vi "LakeShore336_Controller_v2.vi"() -> ()   [LabVIEW 2020]
uses:
  LabVIEW 2020/instr.lib/Lake Shore 336/Public/Data/Sensor Data (Single Reading).vi
  Users/labpc/Documents/ProbeStation Users Data/Yi Hsun/Yi Hsun LabView Program/SubVIs/Lake Shore 336/Lake Shore 336.lvlib
panel:
  in  "Shield \nRate (D) (%)":dbl format="%.1f"
  in  "Shield \nReset (I)":dbl=20.0 format="%.1f"
  in  "Shield\nGain (P)":dbl=50.0 format="%.1f"
  in  "Stage \nRate (D) (%)":dbl format="%.1f"
  in  "Stage \nReset (I)":dbl=20.0 format="%.1f"
  in  "Stage \nGain (P)":dbl=50.0 format="%.1f"
  out "Shield\nHeater1\nON? (Red)":bool
  out "Stage \nHeater2 \nON? (Red)":bool
  out "Out1 Range":u16(ring) items=["Off", "Low (On)", "Medium", "High"]
  out "Out2 Range":u16(ring) items=["Off", "Low (On)", "Medium", "High"]
  out "Output Sel":u16(ring)=2 items=["1"=1, "2"=2]
  out "Input Sel":u16(ring) items=["A", "B", "C", "D"]
  in  "Run Setup?\nStage Heater":bool
  in  "Stage Setpoint \nRamping Enable":bool=TRUE
  out "Out1 Heater %":dbl format="%.1f"
  out "InB Temp":dbl format="%.4f"
  out "Out1 Setpoint":dbl format="%.5f"
  out "Out2 Heater %":dbl format="%.1f"
  out "InA Temp":dbl format="%.4f"
  out "Out2 Setpoint":dbl format="%.5f"
  out "Out2 Diff. (D)":dbl format="%.1f"
  out "Out2 Int. (I)":dbl=20.0 format="%.1f"
  out "Out2 Prop. (P)":dbl=50.0 format="%.1f"
  out "Out1 Diff. (D)":dbl format="%.1f"
  out "Out1 Int. (I)":dbl=20.0 format="%.1f"
  out "Out1 Prop. (P)":dbl=50.0 format="%.1f"
  out "Probe Arm Temperature":dbl format="%.4f"
  out "Temp vs Time 3":cluster{"Y":dbl[], "Y":dbl[]}[](graph)
  out "Stage Setpoint vs Input X Temp 3":cluster{"Sensor Data":dbl}[](graph)
  out "Shield  vs Time 2":cluster{"Y":dbl[], "Y":dbl[]}[](graph)
  out "Shield Setpoint vs Input X Temp 2":cluster{"Setpoint":dbl, "Sensor Data":dbl}[](graph)
  out "Input Sel 2":u16(ring) items=["A", "B", "C", "D"]
  out "Output Sel2":u16(ring)=2 items=["1"=1, "2"=2]
  in  "Run Setup?\nRadiation Heater":bool
  in  "Shield Heater\nRange":u16(ring) items=["Off", "Low (On)", "Medium", "High"]
  in  "Shield Ramp\nRate (K/min)":dbl=5.0 format="%.1f"
  in  "Shield Setpoint (K)":dbl=290.0 format="%.5f"
  in  "Shield Setpoint \nRamping Enable":bool=TRUE
  out "Stage Temp vs Time":cluster{"Y":dbl[], "Y":dbl[]}[](graph)
  out "Stage Setpoint vs Input X Temp":cluster{"Setpoint":dbl, "Sensor Data":dbl}[](graph)
  in  "Stage Heater\nRange":u16(ring) items=["Off", "Low (On)", "Medium", "High"]
  in  "Stage Ramp\nRate (K/min)":dbl=5.0 format="%.1f"
  in  "Stage Setpoint (K)":dbl=290.0 format="%.5f"
  out "Out4 Setpoint":dbl format="%.5f"
  out "Out3 Setpoint":dbl format="%.5f"
  in  "Sampling (ms) [Min 300ms]":u32=300
  in  "stop":bool
  in  "Serial Configuration 2":T1={"Baud Rate"=57600, "Parity"=1, "Data Bits"=7, "Stop Bits"=10, "Flow Control"=0} {"Flow Control" items=["None", "XON/XOFF", "RTS/CTS", "XON/XOFF & RTS/CTS", "DTR/DSR", "XON/XOFF & DTR/DSR"]; "Stop Bits" items=["1.0"=10, "1.5"=15, "2.0"=20]; "Data Bits" items=["7"=7, "8"=8]; "Parity" items=["None", "Odd", "Even", "Mark", "Space"]; "Baud Rate" items=["300"=300, "600"=600, "1200"=1200, "2400"=2400, "4800"=4800, "9600"=9600, "19200"=19200, "38400"=38400, "57600"=57600]}
  in  "LakeShore 336 esource name":refnum<visa-resource-name>="GPIB0::12::INSTR"
  # "Radiation Shield Controller"
  # "Stage Controller"
  # "Click to run sheild parameter setup -->"
  # "Stage Heater Parameters"
  # "Stage PID Parameters"
  # "Shield Heater Parameters"
  # "Shield PID Parameters"
  # "Stage Heater\nStatus"
  # "Shield Heater\nStatus"
  # "Click to run stage parameter setup -->"
  # "PID\nReadout"
  # "PID\nReadout"
  # "Input & Output\nInformation"
  # "Input Selections\nA - Sample stage,     B - Rad Shield,    \nC - Arm,    D - Disabled"
  # "Output Selections\n1 - Rad Shield,     2 - Sample Stage"
  # "Probe\nArm\nMonitor"
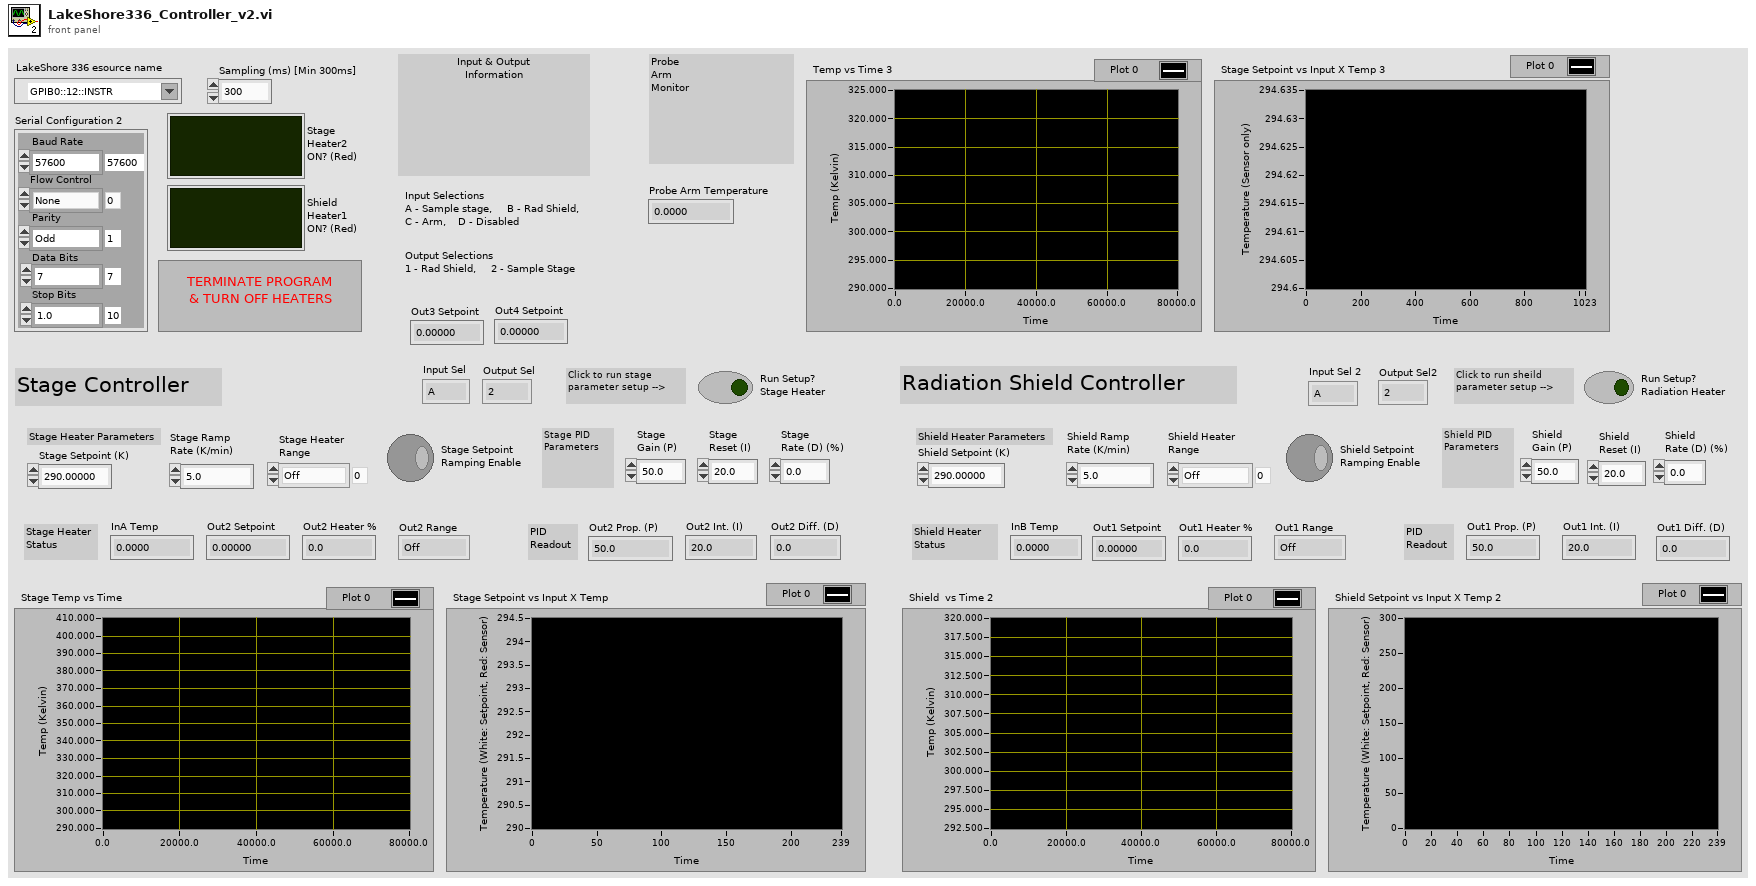
[diagram p1: front panel]
types:
  T1 = cluster{"Baud Rate":u32, "Parity":u16, "Data Bits":u16, "Stop Bits":u16, "Flow Control":u16}
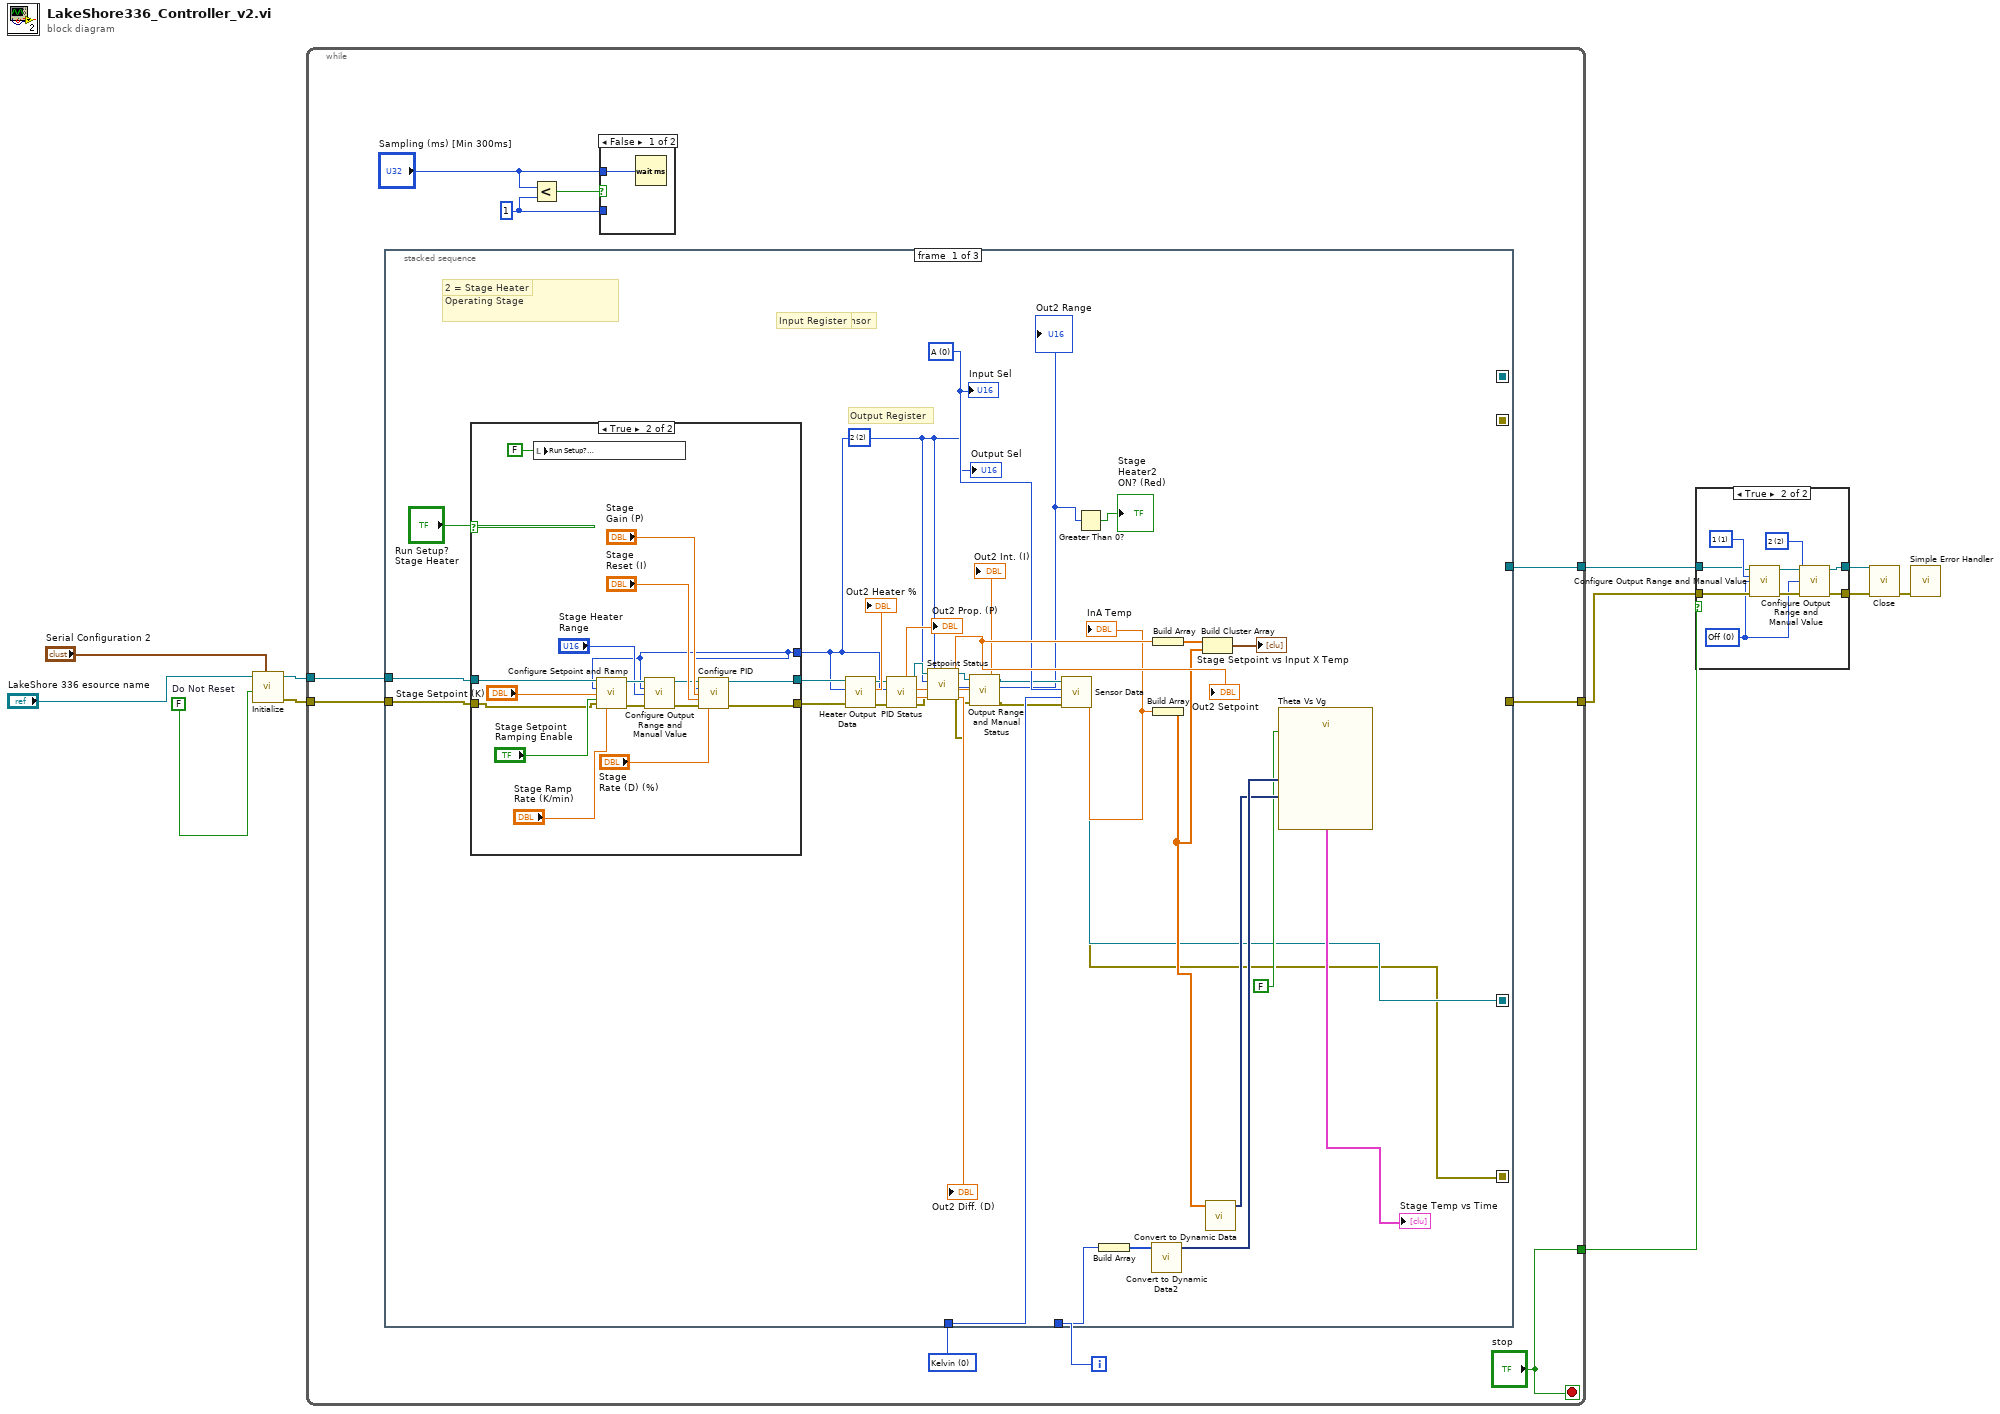
[diagram p0: block diagram]
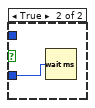
[diagram p3: hidden frame]
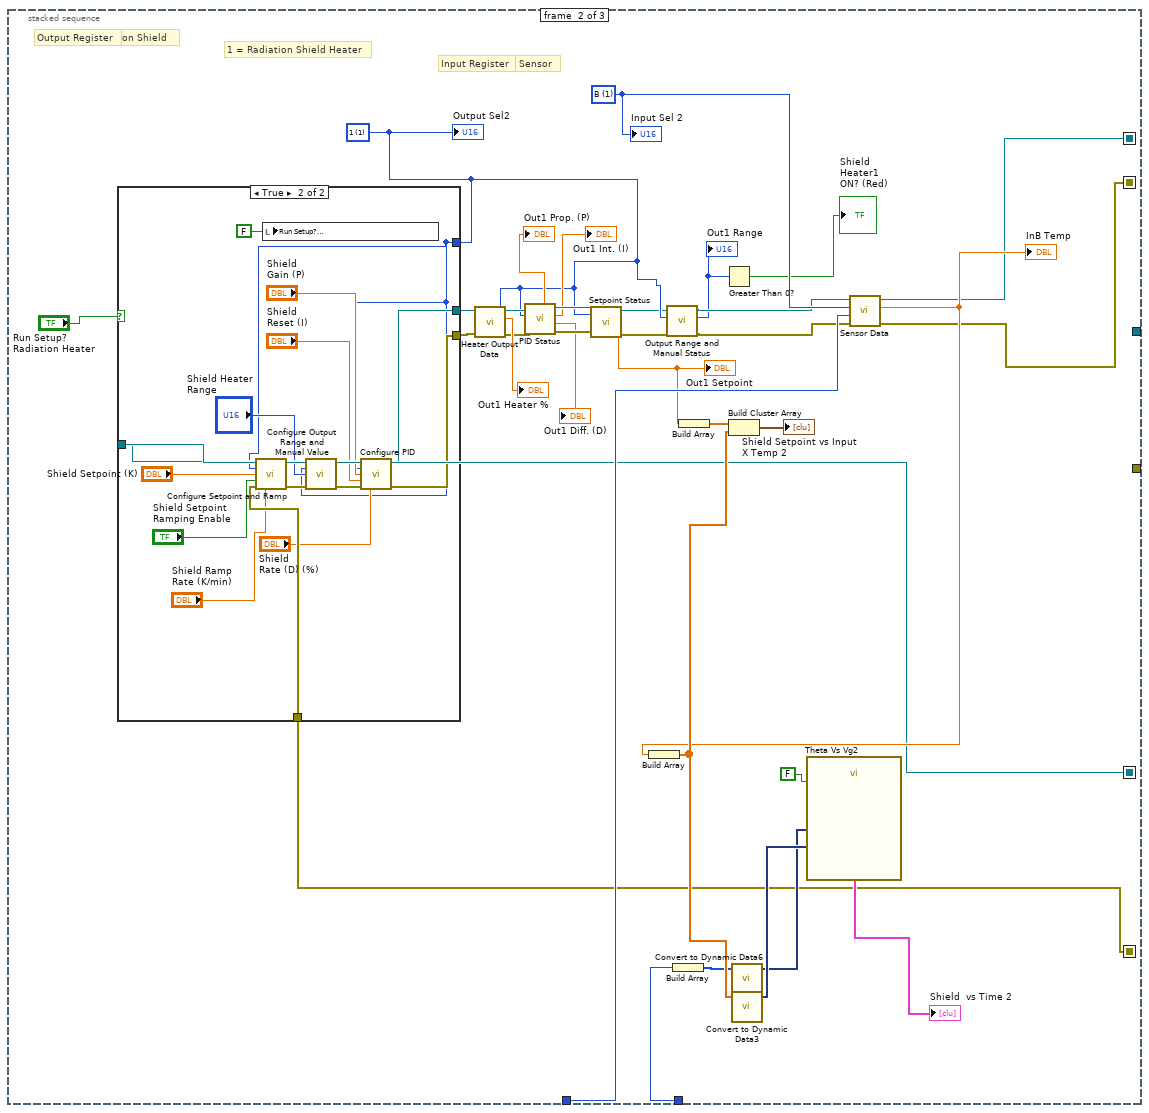
[diagram p5: hidden frame]
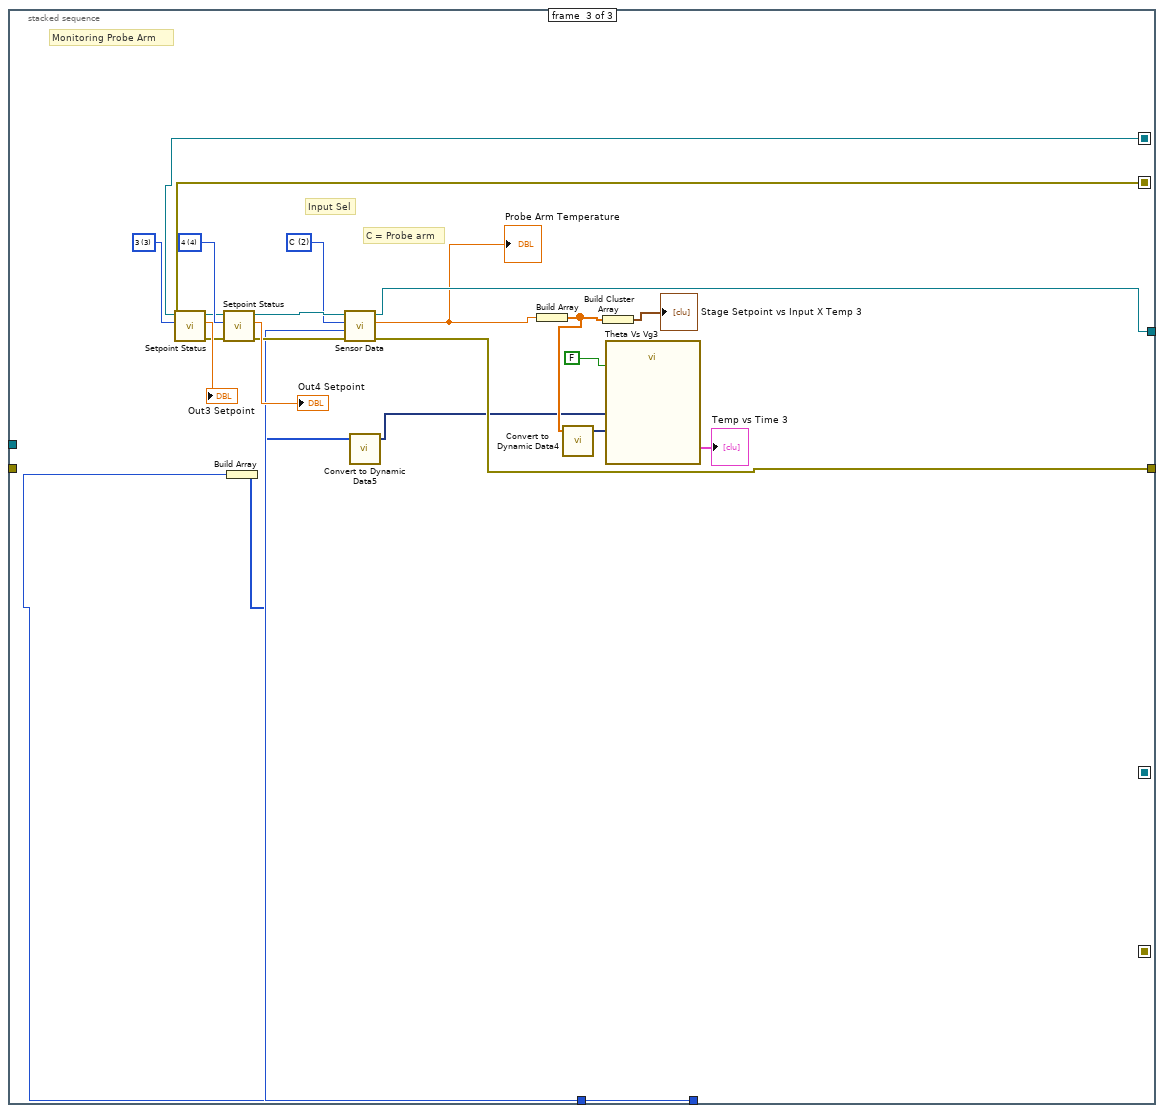
[diagram p7: hidden frame]
diagram:
  w9 = FALSE  # Do Not Reset
  n1 = call "Initialize.vi"("Serial Configuration"="Serial Configuration 2", "Reset (True)"=w9, "VISA resource name"="LakeShore 336 esource name") -> ("error out"=w6:errorcluster, "VISA resource name out"=w7:refnum<visa-resource-name>)  [unwired: 7 in]
  n2 = while {
    tunnel: w7 -> [w21]
    tunnel: w6 -> [w20]
    tunnel: [w19] -> w4
    tunnel: [w18] -> w2
    tunnel: ["stop"] -> w5
    i -> [w14]
    stop <- "stop" stop-if-true
    w13 = u16 0 items=["Kelvin", "Celsius", "Sensor Units"] ("Data Source (0:Kelvin)")
    w16 = u32 1 ("y")
    n3 = stacked-sequence {
      seq-local: [w42 _ _] -> [_ w98 _]
      seq-local: [w41 _ _] -> [_ w97 _]
      seq-local: [_ w96 _] -> [_ _ w147]
      seq-local: [_ w95 _] -> [_ _ w146]
      tunnel: w21 -> [w57 _ _]
      tunnel: w20 -> [w56 _ _]
      tunnel: [_ _ w143] -> w19
      tunnel: [_ _ w142] -> w18
      tunnel: w14 -> [w45 w102 w134]
      tunnel: w13 -> [w43 w104 w138]
      frame #0 {
        w47 = u16 0 items=["A", "B", "C", "D"] ("Input (0:A)\nA - Sample\nB - Rad Shield\nC - Arm\nD - Disabled")
        w26 = u16 2 items=["1"=1, "2"=2] ("Heater Output (1:1)")
        # "A = Stage Sensor"
        # "2 = Stage Heater"
        # "Input Register"
        # "Output Register"
        # "Operating Stage"
        n4 = case shown="True" "Run Setup?\nStage Heater" {
          tunnel: w57 -> [w60 w71]
          tunnel: w56 -> [w59 w70]
          tunnel: [w60 w61] -> w40
          tunnel: [w59 w62] -> w39
          tunnel: w26 -> [_ w65]
          frame False {
          }
          frame True {
            n5 = local write "Run Setup?\nStage Heater"(FALSE ("Run Stage Heater Setup?\nOff / On")) -> ()
            n6 = call "Configure Setpoint and Ramp.vi"("VISA resource name"=w71, "Output's Control Loop (1:1)"=w65, "Setpoint (0.00000)"="Stage Setpoint (K)", "Setpoint Ramping \nEnable (F: Off)"="Stage Setpoint \nRamping Enable", "error in (no error)"=w70, "Ramp Rate (0.0)"="Stage Ramp\nRate (K/min)") -> ("VISA resource name out"=w74:refnum<visa-resource-name>, "error out"=w73:errorcluster)  [unwired: 8 in]
            n7 = call "Configure Output Range and Manual Value.vi"("VISA resource name"=w74, "Output (1:1)"=w65, "Range (0:Off)"="Stage Heater\nRange", "error in (no error)"=w73) -> ("VISA resource name out"=w64:refnum<visa-resource-name>, "error out"=w63:errorcluster)  [unwired: 10 in]
            n8 = call "Configure PID.vi"("VISA resource name"=w64, "Output's Control Loop (1:1)"=w65, "Gain (P) (50.0)"="Stage \nGain (P)", "Reset (I) (20.0)"="Stage \nReset (I)", "error in (no error)"=w63, "Rate (D) (0.0 %)"="Stage \nRate (D) (%)") -> ("VISA resource name out"=w61:refnum<visa-resource-name>, "error out"=w62:errorcluster)  [unwired: 8 in]
          }
        }
        n9 = call "Heater Output Data.vi"("error in (no error)"=w39, "Heater Output (1:1)"=w26, "VISA resource name"=w40) -> ("error out"=w36:errorcluster, "Output Value"=→"Out2 Heater %":dbl, "VISA resource name out"=w37:refnum<visa-resource-name>)  [unwired: 6 in]
        n10 = call "PID Status.vi"("error in (no error)"=w36, "Output's Control Loop (1:1)"=w26, "VISA resource name"=w37) -> ("error out"=w32:errorcluster, "Rate (D)"=→"Out2 Diff. (D)":dbl, "Reset (I)"=→"Out2 Int. (I)":dbl, "VISA resource name out"=w31:refnum<visa-resource-name>, "Gain (P)"=→"Out2 Prop. (P)":dbl)  [unwired: 4 in]
        n11 = call "Setpoint Status.vi"("error in (no error)"=w32, "Output (1:1)"=w26, "VISA resource name"=w31) -> ("error out"=w29:errorcluster, "Setpoint"=w54:dbl, "VISA resource name out"=w30:refnum<visa-resource-name>)  [unwired: 6 in]
        "Out2 Setpoint" <- w54
        n12 = call "Output Range and Manual Status.vi"("error in (no error)"=w29, "Output (1:1)"=w26, "VISA resource name"=w30) -> ("error out"=w27:errorcluster, "Range (0:Off)"=w25:u16, "VISA resource name out"=w28:refnum<visa-resource-name>)  [unwired: 5 in, 1 out]
        "Out2 Range" <- w25
        n13 = call-poly "Sensor Data.vi"("error in (no error)"=w27, "Data Source (0:Kelvin)"=w43, "Input (0:A)"=w47, "VISA resource name"=w28) -> ("error out"=w41:errorcluster, "Sensor Data"=w50:dbl, "VISA resource name out"=w42:refnum<visa-resource-name>)  [unwired: 5 in]
        "InA Temp" <- w50
        n14 = Greater Than 0?(x=w25) -> (x > 0?=→"Stage \nHeater2 \nON? (Red)":bool)
        n15 = Build Array(w45) -> (w44:i32[])
        n16 = call "Convert to Dynamic Data2"("Array"=w44) -> ("Dynamic Data Type"=w52:dynamicdata)  [unwired: 3 in]
        n17 = Build Array(w54) -> (w55:dbl[])
        n18 = Build Array(w50) -> (w53:dbl[])
        n19 = Build Cluster Array(w55, w53) -> (→"Stage Setpoint vs Input X Temp":cluster{"Setpoint":dbl, "Sensor Data":dbl}[])
        n20 = call "Convert to Dynamic Data"("Array"=w53) -> ("Dynamic Data Type"=w51:dynamicdata)  [unwired: 3 in]
        n21 = call "Theta Vs Vg"("Reset"=FALSE, "Y Input"=w51, "X Input"=w52) -> ("XY Graph"=→"Stage Temp vs Time":cluster{"X":dbl[], "Y":dbl[]}[])  [unwired: 7 in, 1 out]
        "Input Sel" <- w47
        "Output Sel" <- w26
      }
      frame #1 {
        w111 = u16 1 items=["A", "B", "C", "D"] ("Input (0:A)\nA - Sample\nB - Rad Shield\nC - Arm\nD - Disabled")
        w84 = u16 1 items=["1"=1, "2"=2] ("Heater Output (1:1)")
        # "B = Radiation Sensor"
        # "Input Register"
        # "1 = Radiation Shield Heater"
        # "Output Register"
        # "Operating Radiation Shield"
        n22 = case shown="True" "Run Setup?\nRadiation Heater" {
          tunnel: w98 -> [w114 w131]
          tunnel: w97 -> [w113 w130]
          tunnel: [w114 w121] -> w93
          tunnel: [w113 w119] -> w92
          tunnel: w84 -> [_ w115]
          frame False {
          }
          frame True {
            n23 = call "Configure Setpoint and Ramp.vi"("VISA resource name"=w131, "Output's Control Loop (1:1)"=w115, "Setpoint (0.00000)"="Shield Setpoint (K)", "Setpoint Ramping \nEnable (F: Off)"="Shield Setpoint \nRamping Enable", "error in (no error)"=w130, "Ramp Rate (0.0)"="Shield Ramp\nRate (K/min)") -> ("VISA resource name out"=w128:refnum<visa-resource-name>, "error out"=w129:errorcluster)  [unwired: 8 in]
            n24 = local write "Run Setup?\nRadiation Heater"(FALSE ("Run Setup?\nRadiation Heater")) -> ()
            n25 = call "Configure Output Range and Manual Value.vi"("VISA resource name"=w128, "Output (1:1)"=w115, "Range (0:Off)"="Shield Heater\nRange", "error in (no error)"=w129) -> ("VISA resource name out"=w122:refnum<visa-resource-name>, "error out"=w120:errorcluster)  [unwired: 10 in]
            n26 = call "Configure PID.vi"("VISA resource name"=w122, "Output's Control Loop (1:1)"=w115, "Gain (P) (50.0)"="Shield\nGain (P)", "Reset (I) (20.0)"="Shield \nReset (I)", "error in (no error)"=w120, "Rate (D) (0.0 %)"="Shield \nRate (D) (%)") -> ("VISA resource name out"=w121:refnum<visa-resource-name>, "error out"=w119:errorcluster)  [unwired: 8 in]
          }
        }
        n27 = call "Heater Output Data.vi"("error in (no error)"=w92, "Heater Output (1:1)"=w84, "VISA resource name"=w93) -> ("error out"=w91:errorcluster, "Output Value"=→"Out1 Heater %":dbl, "VISA resource name out"=w89:refnum<visa-resource-name>)  [unwired: 6 in]
        n28 = call "PID Status.vi"("error in (no error)"=w91, "Output's Control Loop (1:1)"=w84, "VISA resource name"=w89) -> ("error out"=w90:errorcluster, "Rate (D)"=→"Out1 Diff. (D)":dbl, "Reset (I)"=→"Out1 Int. (I)":dbl, "VISA resource name out"=w88:refnum<visa-resource-name>, "Gain (P)"=→"Out1 Prop. (P)":dbl)  [unwired: 4 in]
        n29 = call "Setpoint Status.vi"("error in (no error)"=w90, "Output (1:1)"=w84, "VISA resource name"=w88) -> ("error out"=w82:errorcluster, "Setpoint"=w99:dbl, "VISA resource name out"=w83:refnum<visa-resource-name>)  [unwired: 6 in]
        "Out1 Setpoint" <- w99
        n30 = call "Output Range and Manual Status.vi"("error in (no error)"=w82, "Output (1:1)"=w84, "VISA resource name"=w83) -> ("error out"=w80:errorcluster, "Range (0:Off)"=w79:u16, "VISA resource name out"=w81:refnum<visa-resource-name>)  [unwired: 5 in, 1 out]
        "Out1 Range" <- w79
        n31 = Build Array(w102) -> (w101:i32[])
        n32 = Build Array(w99) -> (w110:dbl[])
        n33 = Greater Than 0?(x=w79) -> (x > 0?=→"Shield\nHeater1\nON? (Red)":bool)
        n34 = call "Convert to Dynamic Data6"("Array"=w101) -> ("Dynamic Data Type"=w100:dynamicdata)  [unwired: 3 in]
        n35 = call-poly "Sensor Data.vi"("error in (no error)"=w80, "Data Source (0:Kelvin)"=w104, "Input (0:A)"=w111, "VISA resource name"=w81) -> ("error out"=w95:errorcluster, "Sensor Data"=w103:dbl, "VISA resource name out"=w96:refnum<visa-resource-name>)  [unwired: 5 in]
        "InB Temp" <- w103
        n36 = Build Array(w103) -> (w105:dbl[])
        n37 = Build Cluster Array(w110, w105) -> (→"Shield Setpoint vs Input X Temp 2":cluster{"Setpoint":dbl, "Sensor Data":dbl}[])
        n38 = call "Convert to Dynamic Data3"("Array"=w105) -> ("Dynamic Data Type"=w109:dynamicdata)  [unwired: 3 in]
        n39 = call "Theta Vs Vg2"("Reset"=FALSE, "Y Input"=w109, "X Input"=w100) -> ("XY Graph"=→"Shield  vs Time 2":cluster{"X":dbl[], "Y":dbl[]}[])  [unwired: 7 in, 1 out]
        "Output Sel2" <- w84
        "Input Sel 2" <- w111
      }
      frame #2 {
        w139 = u16 2 items=["A", "B", "C", "D"] ("Input (0:A)")
        w149 = u16 4 items=["1"=1, "2"=2, "3"=3, "4"=4] ("Output (1:1)")
        w148 = u16 3 items=["1"=1, "2"=2, "3"=3, "4"=4] ("Output (1:1)")
        # "C = Probe arm"
        # "Input Sel"
        # "Monitoring Probe Arm"
        n40 = call "Setpoint Status.vi"("error in (no error)"=w146, "Output (1:1)"=w148, "VISA resource name"=w147) -> ("error out"=w144:errorcluster, "Setpoint"=→"Out3 Setpoint":dbl, "VISA resource name out"=w145:refnum<visa-resource-name>)  [unwired: 6 in]
        n41 = call "Setpoint Status.vi"("error in (no error)"=w144, "Output (1:1)"=w149, "VISA resource name"=w145) -> ("error out"=w140:errorcluster, "Setpoint"=→"Out4 Setpoint":dbl, "VISA resource name out"=w141:refnum<visa-resource-name>)  [unwired: 6 in]
        n42 = Build Array(w134) -> (w133:i32[])
        n43 = call-poly "Sensor Data.vi"("error in (no error)"=w140, "Data Source (0:Kelvin)"=w138, "Input (0:A)"=w139, "VISA resource name"=w141) -> ("error out"=w142:errorcluster, "Sensor Data"=w137:dbl, "VISA resource name out"=w143:refnum<visa-resource-name>)  [unwired: 5 in]
        "Probe Arm Temperature" <- w137
        n44 = call "Convert to Dynamic Data5"("Array"=w133) -> ("Dynamic Data Type"=w132:dynamicdata)  [unwired: 3 in]
        n45 = Build Array(w137) -> (w135:dbl[])
        n46 = call "Convert to Dynamic Data4"("Array"=w135) -> ("Dynamic Data Type"=w154:dynamicdata)  [unwired: 3 in]
        n47 = Build Cluster Array(w135) -> (→"Stage Setpoint vs Input X Temp 3":cluster{"Sensor Data":dbl}[])
        n48 = call "Theta Vs Vg3"("Reset"=FALSE, "Y Input"=w154, "X Input"=w132) -> ("XY Graph"=→"Temp vs Time 3":cluster{"X":dbl[], "Y":dbl[]}[])  [unwired: 7 in, 1 out]
      }
    }
    n49 = Less?(x="Sampling (ms) [Min 300ms]", y=w16) -> (x < y?=w17:bool)
    n50 = case shown="False" w17 {
      tunnel: w16 -> [_ w23]
      tunnel: "Sampling (ms) [Min 300ms]" -> [w22 _]
      frame False {
        n51 = Wait (ms)(milliseconds to wait=w22) -> ()  [unwired: 1 out]
      }
      frame True {
        n52 = Wait (ms)(milliseconds to wait=w23) -> ()  [unwired: 1 out]
      }
    }
  }
  n53 = case shown="True" w5 {
    tunnel: w4 -> [w156 w163]
    tunnel: [w156 w161] -> w3
    tunnel: w2 -> [w155 w160]
    tunnel: [w155 w158] -> w1
    frame False {
    }
    frame True {
      w157 = u16 0 items=["Off", "Low (On)", "Medium", "High"] ("Range (0:Off)")
      w165 = u16 2 items=["1"=1, "2"=2, "3"=3, "4"=4] ("Output (1:1)")
      w164 = u16 1 items=["1"=1, "2"=2, "3"=3, "4"=4] ("Output (1:1)")
      n54 = call "Configure Output Range and Manual Value.vi"("VISA resource name"=w163, "Output (1:1)"=w164, "Range (0:Off)"=w157, "error in (no error)"=w160) -> ("VISA resource name out"=w162:refnum<visa-resource-name>, "error out"=w159:errorcluster)  [unwired: 10 in]
      n55 = call "Configure Output Range and Manual Value.vi"("VISA resource name"=w162, "Output (1:1)"=w165, "Range (0:Off)"=w157, "error in (no error)"=w159) -> ("VISA resource name out"=w161:refnum<visa-resource-name>, "error out"=w158:errorcluster)  [unwired: 10 in]
    }
  }
  n56 = call "Close.vi"("error in (no error)"=w1, "VISA resource name"=w3) -> ("error out"=w10:errorcluster)  [unwired: 9 in]
  n57 = call <vilib>:"Simple Error Handler.vi"("error in (no error)"=w10) -> ()  [unwired: 4 in, 5 out]
